vi "Log Data.vi"(8 "error in (no error)":errorcluster, 9 "Data":waveform(dbl)[](array[waveform]), 11 "Logger in.lvclass":refnum<class "Logger.lvclass">) -> (0 "error out":errorcluster, 1 "Buffer":i32, 2 "Files Sent":i32, 3 "Logger out.lvclass":refnum<class "Logger.lvclass">, 4 "file path out":path)   [LabVIEW 2024, in "Logger.lvclass"]
uses:
  Logger.lvclass
  Logger.lvclass/Logger.ctl
  <vilib>/Skyline/TestMonitor/Test Result/NI SystemLink Test Result.lvclass/NI SystemLink Test Result.ctl
  <vilib>/Skyline/File/HTTP/Send File HTTP.vi
  <vilib>/Skyline/TestMonitor/Test Result/Update Test Result (Single).vi
  <vilib>/Skyline/File/File/NI Skyline File.lvclass
  <vilib>/Skyline/Configuration/Configuration AMQP_class/NI Skyline Configuration AMQP.lvclass
  <vilib>/Skyline/TestMonitor/Test Result/NI SystemLink Test Result.lvclass
  <vilib>/Skyline/File/HTTP/NI Skyline File HTTP.lvclass
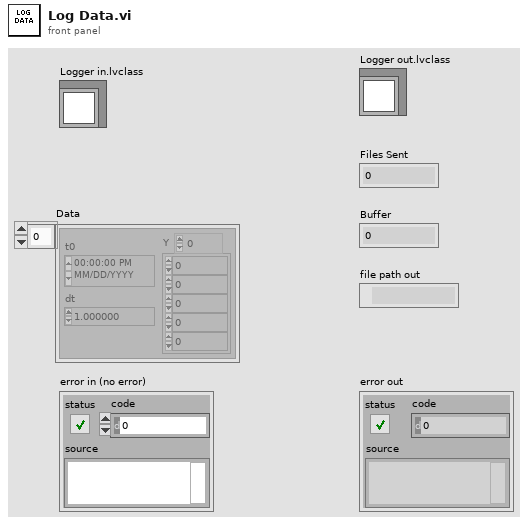
[diagram p1: front panel]
types:
  T1 = enum16{"open", "open or create", "create or replace", "create", "open (read-only)"}
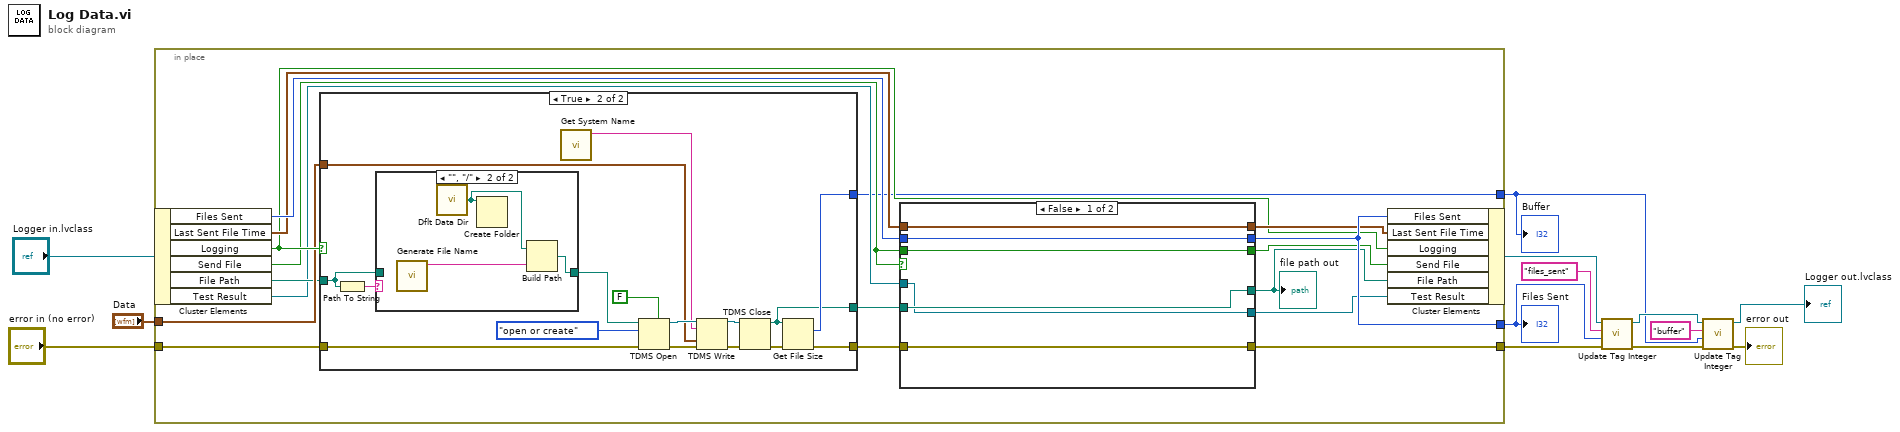
[diagram p0: block diagram]
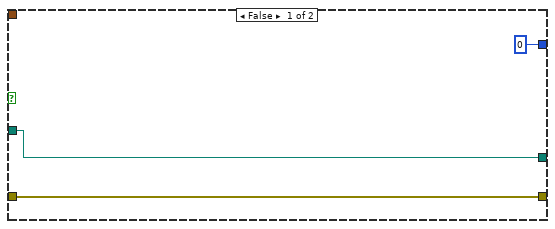
[diagram p2: hidden frame]
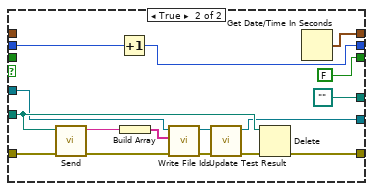
[diagram p4: hidden frame]
diagram:
  n1 = in-place {
    in-place-border: [w29] -> w8
    in-place-border: [w20] -> w9
    in-place-border: "error in (no error)" -> [w22]
    in-place-border: "Data" -> [w25]
    in-place-border: [w14] -> w2
    n2 = in-place-cluster #1("Logger in.lvclass") -> ("Files Sent"=w30:i32, "Last Sent File Time"=w27:timestamp, "Logging"=w26:bool, "Send File"=w18:bool, "File Path"=w24:path, "Test Result"=w16:refnum<class "NI SystemLink Test Result.lvclass">)
    n3 = case shown="True" w26 {
      tunnel: w25 -> [_ w46]
      tunnel: w24 -> [w33 w36]
      tunnel: [w33 w40] -> w23
      tunnel: w22 -> [w32 w42]
      tunnel: [w32 w38] -> w21
      tunnel: [i64 0 ("size (in bytes)") w41] -> w14
      frame False {
      }
      frame True {
        n4 = Path To String(path=w36) -> (string=w35:string)
        n5 = case shown="\"\", \"/\"" w35 {
          tunnel: [w50 w52] -> w37
          tunnel: w36 -> [w50 _]
          frame "False", Default {
          }
          frame "", "/" {
            n6 = call "Generate File Name.vi"() -> ("file name"=w53:string)  [unwired: 11 in]
            n7 = call <vilib>:"Dflt Data Dir.vi"() -> ("App:Default Data Directory"=w51:path)
            n8 = Create Folder(path (use dialog)=w51) -> ()  [unwired: 2 in, 3 out]
            n9 = Build Path(base path=w51, name or relative path=w53) -> (appended path=w52:path)
          }
        }
        n10 = call "Get System Name.vi"() -> ("name"=w43:string)  [unwired: 11 in]
        n11 = TDMS Open(5:FALSE ("create index file? (T)"), 8:w42, 10:T1."open or create" ("operation (0:open)"), 11:w37) -> (0:w47:errorcluster, 3:w48:refnum<k34>)  [unwired: 3 in]
        n12 = TDMS Write(0:w48, 5:w43, 9:w46, 11:w47) -> (4:w44:refnum<k34>, 15:w45:errorcluster)  [unwired: 2 in, 2 out]
        n13 = TDMS Close(8:w45, 11:w44) -> (0:w39:errorcluster, 3:w40:path)
        n14 = Get File Size(file=w40, error in=w39) -> (size (in bytes)=w41:i64, 0:w38:errorcluster)  [unwired: 1 out]
      }
    }
    n15 = case shown="False" w18 {
      tunnel: w30 -> [w59 w75]
      tunnel: [w59 w74] -> w29
      tunnel: [w58 w73] -> w28
      tunnel: w27 -> [w58 _]
      tunnel: [w57 w70] -> w20
      tunnel: w21 -> [w57 w72]
      tunnel: w23 -> [w56 w69]
      tunnel: [w56 path "" ("file path out")] -> w19
      tunnel: w18 -> [w55 _]
      tunnel: [w55 FALSE ("Send File")] -> w17
      tunnel: w16 -> [w54 w66]
      tunnel: [w54 w61] -> w15
      frame False {
      }
      frame True {
        n16 = call-poly <vilib>:"Send.vi"("error in (no error)"=w72, "path"=w69) -> ("error out"=w67:errorcluster, "id"=w65:string)  [unwired: 7 in]
        n17 = Increment(x=w75) -> (x+1=w74:i32)
        n18 = Build Array(w65) -> (w64:string[])
        n19 = call <vilib>:"Write File Ids.vi"("error in (no error)"=w67, "file ids"=w64, "test result in"=w66) -> ("error out"=w62:errorcluster, "test result out"=w63:refnum<class "NI SystemLink Test Result.lvclass">)  [unwired: 7 in]
        n20 = call-poly <vilib>:"Update Test Result.vi"("error in (no error)"=w62, "test result in"=w63) -> ("error out"=w60:errorcluster, "test result out"=w61:refnum<class "NI SystemLink Test Result.lvclass">)  [unwired: 8 in]
        n21 = Delete(path (use dialog)=w69, error in=w60) -> (error out=w70:errorcluster)  [unwired: 3 in, 2 out]
        n22 = Get Date/Time In Seconds() -> (seconds since 1Jan1904=w73:timestamp)
      }
    }
    "file path out" <- w19
    n23 = in-place-cluster #1("Files Sent"=w29, "Last Sent File Time"=w28, "Logging"=w26, "Send File"=w17, "File Path"=w19, "Test Result"=w15) -> (w11:refnum<class "Logger.lvclass">)
  }
  "Files Sent" <- w8
  "Buffer" <- w2
  n24 = call "Update Tag Integer.vi"("error in (no error)"=w9, "Value"=w8, "Tag Path"="files_sent", "Logger in.lvclass"=w11) -> ("error out"=w4:errorcluster, "Logger out.lvclass"=w6:refnum<class "Logger.lvclass">)  [unwired: 6 in]
  n25 = call "Update Tag Integer.vi"("error in (no error)"=w4, "Value"=w2, "Tag Path"="buffer", "Logger in.lvclass"=w6) -> ("error out"=→"error out":errorcluster, "Logger out.lvclass"=→"Logger out.lvclass":refnum<class "Logger.lvclass">)  [unwired: 6 in]
